vi "Constants.vi"() -> ()   [LabVIEW 2013, in "PWM Shared.lvlib"]
doc: "Use this Global VI to access the GUIDs assigned to the page resources of the Custom Device."
uses:
  PWM Shared.lvlib
panel:
  in  "Tab Control":enum32{"GUIDS", "Constants", "Properties"}(tab)=enum."Properties"
  in  "Duty Cycle":string="36b6f866-7f9c-4a3a-a54b-67d62ca87d5a"
  in  "Frequency":string="6c7d90f8-10f7-4005-87f3-4242ea982cd9"
  in  "PWM Write":string="d17e2beb-b952-4967-9a77-9ac6283ecebb"
  in  "PWM Read":string="b16e01b0-f143-4df1-b530-3d2d02e376a4"
  in  "PWM Outputs":string="96b66490-c83d-4717-9412-d019099b8526"
  in  "PWM Inputs":string="4043f575-1c96-4996-88ce-1fbf0167a230"
  in  "PWM":string="9757959c-7257-43ce-849f-f6167fb02ae7"
  in  "Frequency ch":string="Frequency"
  in  "Duty Cycle ch":string="Duty Cycle"
  in  "Write Section":string="Write"
  in  "Read Section":string="Read"
  in  "Device Name":string="PWM"
  in  "Compiled Info":string="Compiled Info"
  in  "Config Info":string="Config Info"
  in  "Timeout":string="Timeout"
  in  "Bitfile Path":string="Bitfile Path"
  in  "FPGA Name":string="FPGA Name"
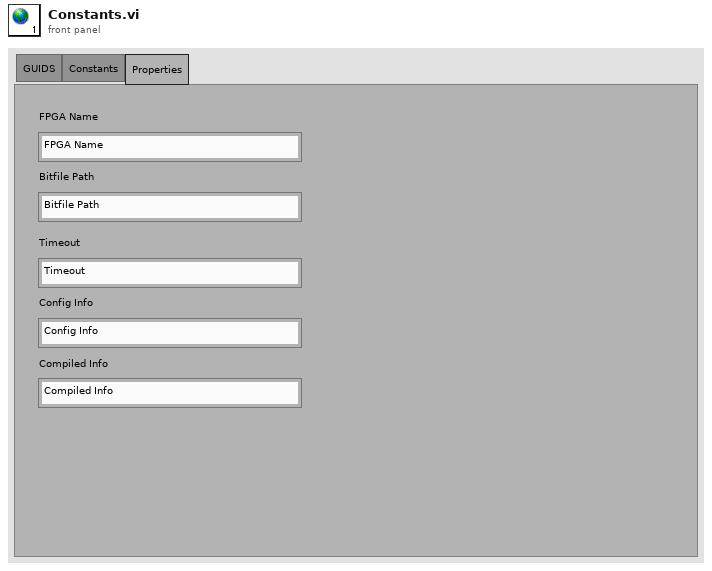
[diagram p1: front panel]
diagram:
